vi "2.Rtde.vi"() -> ()   [LabVIEW 2023]
uses:
  UnderAutomation.UniversalRobots/UnderAutomation.UniversalRobots.lvlib
  C:/Users/fg/Documents/UniversalRobots.vi/LabVIEW_2024/UnderAutomation.UniversalRobots/lib/UnderAutomation.UniversalRobots.dll
  LabVIEW_2024/UnderAutomation.UniversalRobots/lib/UnderAutomation.UniversalRobots.dll
panel:
  out "Rtde":refnum<k24>
  out "UR Robot":refnum<k24>
  out "Connected":bool
  in  "Tab Control":enum32{"Connect to robot", "RTDE data"}(tab)
  in  "Disconnect":bool
  in  "Test":bool
  in  "Key":string
  in  "Licensee":string
  in  "Connect":bool
  in  "IP":string caption="Robot IP Address"
  out "License state":string
  out "Connect error":string
  in  "Speed":dbl(slide) scale=0.0..1.0 scale format="%#_2f"
  out "ActualTcpPose":T1
  out "TargetTcpSpeed":T1
  out "ScriptControlLine":u32
  out "OutputDoubleRegisters.X10":dbl
  out "OutputIntRegisters.X3":i32
  out "OutputIntRegisters.X2":i32
  out "OutputDoubleRegisters.X11":dbl
  out "OutputBitRegisters.X64":bool
  in  "InputIntRegisters.X11":i32
  in  "InputIntRegisters.X10":i32
  in  "Write":bool
  in  "stop":bool
  # "UnderAutomation"
  # "https://underautomation.com/universal-robots"
  # "+"
  # "LabVIEW demo app for remote control and monitoring of your Universal Robots cobot"
  # "Connect to robot"
  # "2. Ensure you have a trial or lifetime valid license"
  # "1. Set UR cobot address"
  # "This is a commercial library, you have a 30-day trial period. But you can use it forever if you buy a perpetual licence for your company (regardless of the number of robot, applications or developers)."
  # "If you have a license :"
  # "2. Connect to the robot"
  # "Output data received from robot"
  # "Output data received from robot"
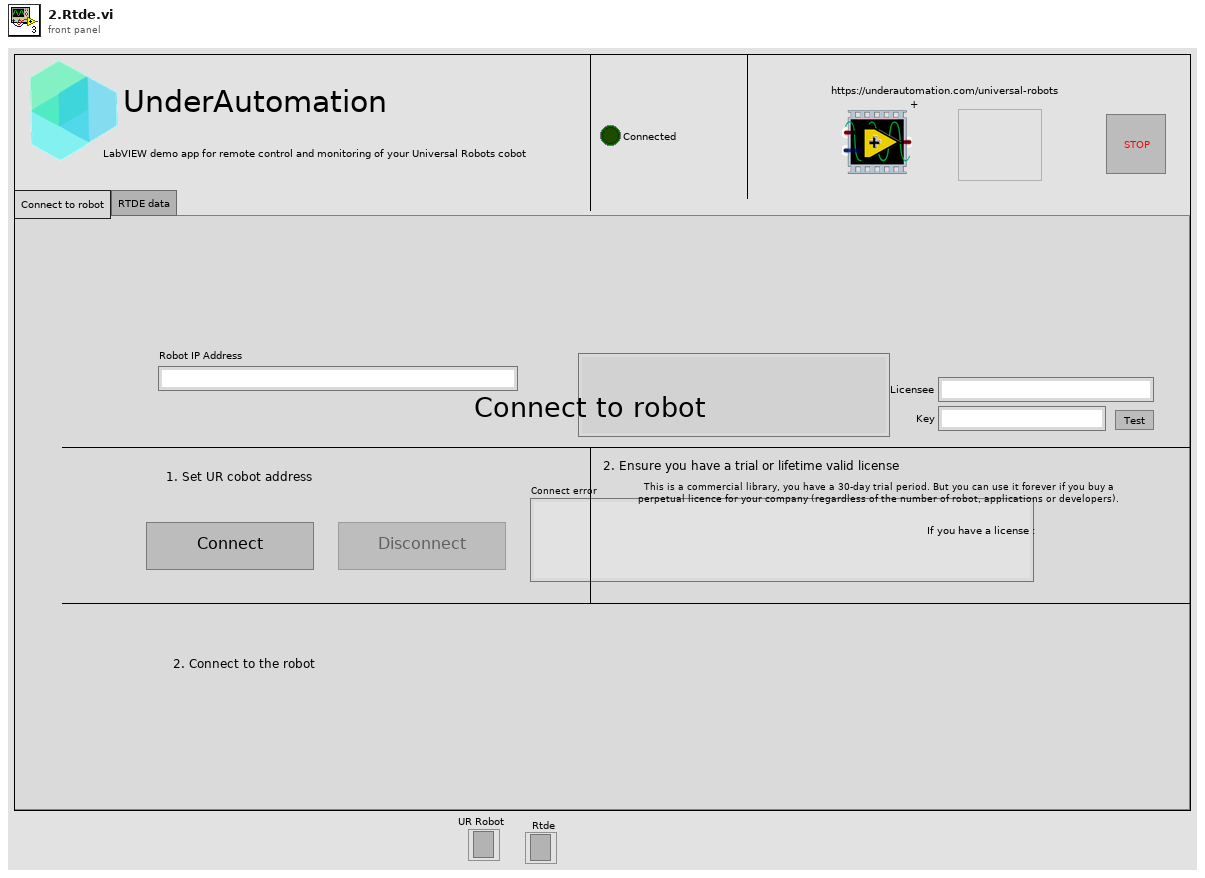
[diagram p1: front panel]
types:
  T1 = cluster{"X":dbl, "Y":dbl, "Z":dbl, "Rx":dbl, "Ry":dbl, "Rz":dbl}
  T2 = cluster{"ConfigurableDigitalOutput":u8, "ConfigurableDigitalOutputMask":u8, "ExternalForceTorque":cluster{"X":dbl, "Y":dbl, "Z":dbl, "Rx":dbl, "Ry":dbl, "Rz":dbl}, "InputBitRegisters":cluster{"X64":bool, "X65":bool, "X66":bool, "X67":bool, "X68":bool, "X69":bool, "X70":bool, "X71":bool, "X72":bool, "X73":bool, "X74":bool, "X75":bool, "X76":bool, "X77":bool, "X78":bool, "X79":bool, "X80":bool, "X81":bool, "X82":bool, "X83":bool, "X84":bool, "X85":bool, "X86":bool, "X87":bool, "X88":bool, "X89":bool, "X90":bool, "X91":bool, "X92":bool, "X93":bool, "X94":bool, "X95":bool, "X96":bool, "X97":bool, "X98":bool, "X99":bool, "X100":bool, "X101":bool, "X102":bool, "X103":bool, "X104":bool, "X105":bool, "X106":bool, "X107":bool, "X108":bool, "X109":bool, "X110":bool, "X111":bool, "X112":bool, "X113":bool, "X114":bool, "X115":bool, "X116":bool, "X117":bool, "X118":bool, "X119":bool, "X120":bool, "X121":bool, "X122":bool, "X123":bool, "X124":bool, "X125":bool, "X126":bool, "X127":bool}, "InputBtRegisters0To31":u32, "InputBtRegisters32To63":u32, "InputDoubleRegisters":cluster{"X0":dbl, "X1":dbl, "X2":dbl, "X3":dbl, "X4":dbl, "X5":dbl, "X6":dbl, "X7":dbl, "X8":dbl, "X9":dbl, "X10":dbl, "X11":dbl, "X12":dbl, "X13":dbl, "X14":dbl, "X15":dbl, "X16":dbl, "X17":dbl, "X18":dbl, "X19":dbl, "X20":dbl, "X21":dbl, "X22":dbl, "X23":dbl, "X24":dbl, "X25":dbl, "X26":dbl, "X27":dbl, "X28":dbl, "X29":dbl, "X30":dbl, "X31":dbl, "X32":dbl, "X33":dbl, "X34":dbl, "X35":dbl, "X36":dbl, "X37":dbl, "X38":dbl, "X39":dbl, "X40":dbl, "X41":dbl, "X42":dbl, "X43":dbl, "X44":dbl, "X45":dbl, "X46":dbl, "X47":dbl}, "InputIntRegisters":cluster{"X0":i32, "X1":i32, "X2":i32, "X3":i32, "X4":i32, "X5":i32, "X6":i32, "X7":i32, "X8":i32, "X9":i32, "X10":i32, "X11":i32, "X12":i32, "X13":i32, "X14":i32, "X15":i32, "X16":i32, "X17":i32, "X18":i32, "X19":i32, "X20":i32, "X21":i32, "X22":i32, "X23":i32, "X24":i32, "X25":i32, "X26":i32, "X27":i32, "X28":i32, "X29":i32, "X30":i32, "X31":i32, "X32":i32, "X33":i32, "X34":i32, "X35":i32, "X36":i32, "X37":i32, "X38":i32, "X39":i32, "X40":i32, "X41":i32, "X42":i32, "X43":i32, "X44":i32, "X45":i32, "X46":i32, "X47":i32}, "SpeedSliderFraction":dbl, "SpeedSliderMask":u32, "StandardAnalogOutput0":dbl, "StandardAnalogOutput1":dbl, "StandardAnalogOutputMask":u8, "StandardAnalogOutputType":u8, "StandardDigitalOutput":u8, "StandardDigitalOutputMask":u8}
  T3 = enum8{"Enabled", "Disabled", "Disabled and Grayed Out"}
  T4 = cluster{"ActualCurrent":cluster{"Base":dbl, "Elbow":dbl, "Shoulder":dbl, "Wrist1":dbl, "Wrist2":dbl, "Wrist3":dbl}, "ActualDigitalInputBits":u64, "ActualDigitalOutputBits":u64, "ActualExecutionTime":dbl, "ActualJointVoltage":cluster{"Base":dbl, "Elbow":dbl, "Shoulder":dbl, "Wrist1":dbl, "Wrist2":dbl, "Wrist3":dbl}, "ActualMainVoltage":dbl, "ActualMomentum":dbl, "ActualQ":cluster{"Base":dbl, "Elbow":dbl, "Shoulder":dbl, "Wrist1":dbl, "Wrist2":dbl, "Wrist3":dbl}, "ActualQd":cluster{"Base":dbl, "Elbow":dbl, "Shoulder":dbl, "Wrist1":dbl, "Wrist2":dbl, "Wrist3":dbl}, "ActualRobotCurrent":dbl, "ActualRobotVoltage":dbl, "ActualTcpForce":cluster{"X":dbl, "Y":dbl, "Z":dbl, "Rx":dbl, "Ry":dbl, "Rz":dbl}, "ActualTcpPose":cluster{"X":dbl, "Y":dbl, "Z":dbl, "Rx":dbl, "Ry":dbl, "Rz":dbl}, "ActualTcpSpeed":cluster{"X":dbl, "Y":dbl, "Z":dbl, "Rx":dbl, "Ry":dbl, "Rz":dbl}, "ActualToolAccelerometer":cluster{"X":dbl, "Y":dbl, "Z":dbl}, "AnalogIOTypes":u32, "ElbowPosition":cluster{"X":dbl, "Y":dbl, "Z":dbl}, "ElbowVelocity":cluster{"X":dbl, "Y":dbl, "Z":dbl}, "Euromap67_24VCurrent":dbl, "Euromap67_24VVoltage":dbl, "Euromap67InputBits":u32, "Euromap67OutputBits":u32, "FTRawWrench":cluster{"X":dbl, "Y":dbl, "Z":dbl, "Rx":dbl, "Ry":dbl, "Rz":dbl}, "InputBitRegisters":cluster{"X64":bool, "X65":bool, "X66":bool, "X67":bool, "X68":bool, "X69":bool, "X70":bool, "X71":bool, "X72":bool, "X73":bool, "X74":bool, "X75":bool, "X76":bool, "X77":bool, "X78":bool, "X79":bool, "X80":bool, "X81":bool, "X82":bool, "X83":bool, "X84":bool, "X85":bool, "X86":bool, "X87":bool, "X88":bool, "X89":bool, "X90":bool, "X91":bool, "X92":bool, "X93":bool, "X94":bool, "X95":bool, "X96":bool, "X97":bool, "X98":bool, "X99":bool, "X100":bool, "X101":bool, "X102":bool, "X103":bool, "X104":bool, "X105":bool, "X106":bool, "X107":bool, "X108":bool, "X109":bool, "X110":bool, "X111":bool, "X112":bool, "X113":bool, "X114":bool, "X115":bool, "X116":bool, "X117":bool, "X118":bool, "X119":bool, "X120":bool, "X121":bool, "X122":bool, "X123":bool, "X124":bool, "X125":bool, "X126":bool, "X127":bool}, "InputBitRegisters0To31":u32, "InputBitRegisters32To63":u32, "InputDoubleRegisters":cluster{"X0":dbl, "X1":dbl, "X2":dbl, "X3":dbl, "X4":dbl, "X5":dbl, "X6":dbl, "X7":dbl, "X8":dbl, "X9":dbl, "X10":dbl, "X11":dbl, "X12":dbl, "X13":dbl, "X14":dbl, "X15":dbl, "X16":dbl, "X17":dbl, "X18":dbl, "X19":dbl, "X20":dbl, "X21":dbl, "X22":dbl, "X23":dbl, "X24":dbl, "X25":dbl, "X26":dbl, "X27":dbl, "X28":dbl, "X29":dbl, "X30":dbl, "X31":dbl, "X32":dbl, "X33":dbl, "X34":dbl, "X35":dbl, "X36":dbl, "X37":dbl, "X38":dbl, "X39":dbl, "X40":dbl, "X41":dbl, "X42":dbl, "X43":dbl, "X44":dbl, "X45":dbl, "X46":dbl, "X47":dbl}, "InputIntRegisters":cluster{"X0":i32, "X1":i32, "X2":i32, "X3":i32, "X4":i32, "X5":i32, "X6":i32, "X7":i32, "X8":i32, "X9":i32, "X10":i32, "X11":i32, "X12":i32, "X13":i32, "X14":i32, "X15":i32, "X16":i32, "X17":i32, "X18":i32, "X19":i32, "X20":i32, "X21":i32, "X22":i32, "X23":i32, "X24":i32, "X25":i32, "X26":i32, "X27":i32, "X28":i32, "X29":i32, "X30":i32, "X31":i32, "X32":i32, "X33":i32, "X34":i32, "X35":i32, "X36":i32, "X37":i32, "X38":i32, "X39":i32, "X40":i32, "X41":i32, "X42":i32, "X43":i32, "X44":i32, "X45":i32, "X46":i32, "X47":i32}, "IOCurrent":dbl, "JointControlOutput":cluster{"Base":dbl, "Elbow":dbl, "Shoulder":dbl, "Wrist1":dbl, "Wrist2":dbl, "Wrist3":dbl}, "JointMode":cluster{"Base":i32, "Elbow":i32, "Shoulder":i32, "Wrist1":i32, "Wrist2":i32, "Wrist3":i32}, "JointTemperatures":cluster{"Base":dbl, "Elbow":dbl, "Shoulder":dbl, "Wrist1":dbl, "Wrist2":dbl, "Wrist3":dbl}, "OutputBitRegisters":cluster{"X64":bool, "X65":bool, "X66":bool, "X67":bool, "X68":bool, "X69":bool, "X70":bool, "X71":bool, "X72":bool, "X73":bool, "X74":bool, "X75":bool, "X76":bool, "X77":bool, "X78":bool, "X79":bool, "X80":bool, "X81":bool, "X82":bool, "X83":bool, "X84":bool, "X85":bool, "X86":bool, "X87":bool, "X88":bool, "X89":bool, "X90":bool, "X91":bool, "X92":bool, "X93":bool, "X94":bool, "X95":bool, "X96":bool, "X97":bool, "X98":bool, "X99":bool, "X100":bool, "X101":bool, "X102":bool, "X103":bool, "X104":bool, "X105":bool, "X106":bool, "X107":bool, "X108":bool, "X109":bool, "X110":bool, "X111":bool, "X112":bool, "X113":bool, "X114":bool, "X115":bool, "X116":bool, "X117":bool, "X118":bool, "X119":bool, "X120":bool, "X121":bool, "X122":bool, "X123":bool, "X124":bool, "X125":bool, "X126":bool, "X127":bool}, "OutputBitRegisters0To31":u32, "OutputBitRegisters32To63":u32, "OutputDoubleRegisters":cluster{"X0":dbl, "X1":dbl, "X2":dbl, "X3":dbl, "X4":dbl, "X5":dbl, "X6":dbl, "X7":dbl, "X8":dbl, "X9":dbl, "X10":dbl, "X11":dbl, "X12":dbl, "X13":dbl, "X14":dbl, "X15":dbl, "X16":dbl, "X17":dbl, "X18":dbl, "X19":dbl, "X20":dbl, "X21":dbl, "X22":dbl, "X23":dbl, "X24":dbl, "X25":dbl, "X26":dbl, "X27":dbl, "X28":dbl, "X29":dbl, "X30":dbl, "X31":dbl, "X32":dbl, "X33":dbl, "X34":dbl, "X35":dbl, "X36":dbl, "X37":dbl, "X38":dbl, "X39":dbl, "X40":dbl, "X41":dbl, "X42":dbl, "X43":dbl, "X44":dbl, "X45":dbl, "X46":dbl, "X47":dbl}, "OutputIntRegisters":cluster{"X0":i32, "X1":i32, "X2":i32, "X3":i32, "X4":i32, "X5":i32, "X6":i32, "X7":i32, "X8":i32, "X9":i32, "X10":i32, "X11":i32, "X12":i32, "X13":i32, "X14":i32, "X15":i32, "X16":i32, "X17":i32, "X18":i32, "X19":i32, "X20":i32, "X21":i32, "X22":i32, "X23":i32, "X24":i32, "X25":i32, "X26":i32, "X27":i32, "X28":i32, "X29":i32, "X30":i32, "X31":i32, "X32":i32, "X33":i32, "X34":i32, "X35":i32, "X36":i32, "X37":i32, "X38":i32, "X39":i32, "X40":i32, "X41":i32, "X42":i32, "X43":i32, "X44":i32, "X45":i32, "X46":i32, "X47":i32}, "Payload":dbl, "PayloadCOG":cluster{"X":dbl, "Y":dbl, "Z":dbl}, "PayloadInertia":cluster{"X":dbl, "Y":dbl, "Z":dbl, "Rx":dbl, "Ry":dbl, "Rz":dbl}, "RobotMode":i32, "RobotStatusBits":u32, "RuntimeState":u32, "SafetyMode":i32, "SafetyStatus":i32, "SafetyStatusBits":u32, "ScriptControlLine":u32, "SpeedScaling":dbl, "StandardAnalogInput0":dbl, "StandardAnalogInput1":dbl, "StandardAnalogOutput0":dbl, "StandardAnalogOutput1":dbl, "TargetCurrent":cluster{"Base":dbl, "Elbow":dbl, "Shoulder":dbl, "Wrist1":dbl, "Wrist2":dbl, "Wrist3":dbl}, "TargetMoment":cluster{"Base":dbl, "Elbow":dbl, "Shoulder":dbl, "Wrist1":dbl, "Wrist2":dbl, "Wrist3":dbl}, "TargetQ":cluster{"Base":dbl, "Elbow":dbl, "Shoulder":dbl, "Wrist1":dbl, "Wrist2":dbl, "Wrist3":dbl}, "TargetQd":cluster{"Base":dbl, "Elbow":dbl, "Shoulder":dbl, "Wrist1":dbl, "Wrist2":dbl, "Wrist3":dbl}, "TargetQdd":cluster{"Base":dbl, "Elbow":dbl, "Shoulder":dbl, "Wrist1":dbl, "Wrist2":dbl, "Wrist3":dbl}, "TargetSpeedFraction":dbl, "TargetTcpPose":cluster{"X":dbl, "Y":dbl, "Z":dbl, "Rx":dbl, "Ry":dbl, "Rz":dbl}, "TargetTcpSpeed":cluster{"X":dbl, "Y":dbl, "Z":dbl, "Rx":dbl, "Ry":dbl, "Rz":dbl}, "TcpForceScalar":dbl, "Timestamp":dbl, "ToolAnalogInput0":dbl, "ToolAnalogInput1":dbl, "ToolAnalogInputTypes":u32, "ToolDigitalOutput0mode":u8, "ToolDigitalOutput1Mode":u8, "ToolMode":u32, "ToolOutputCurrent":dbl, "ToolOutputMode":u8, "ToolOutputVoltage":i32, "ToolTemperature":dbl}
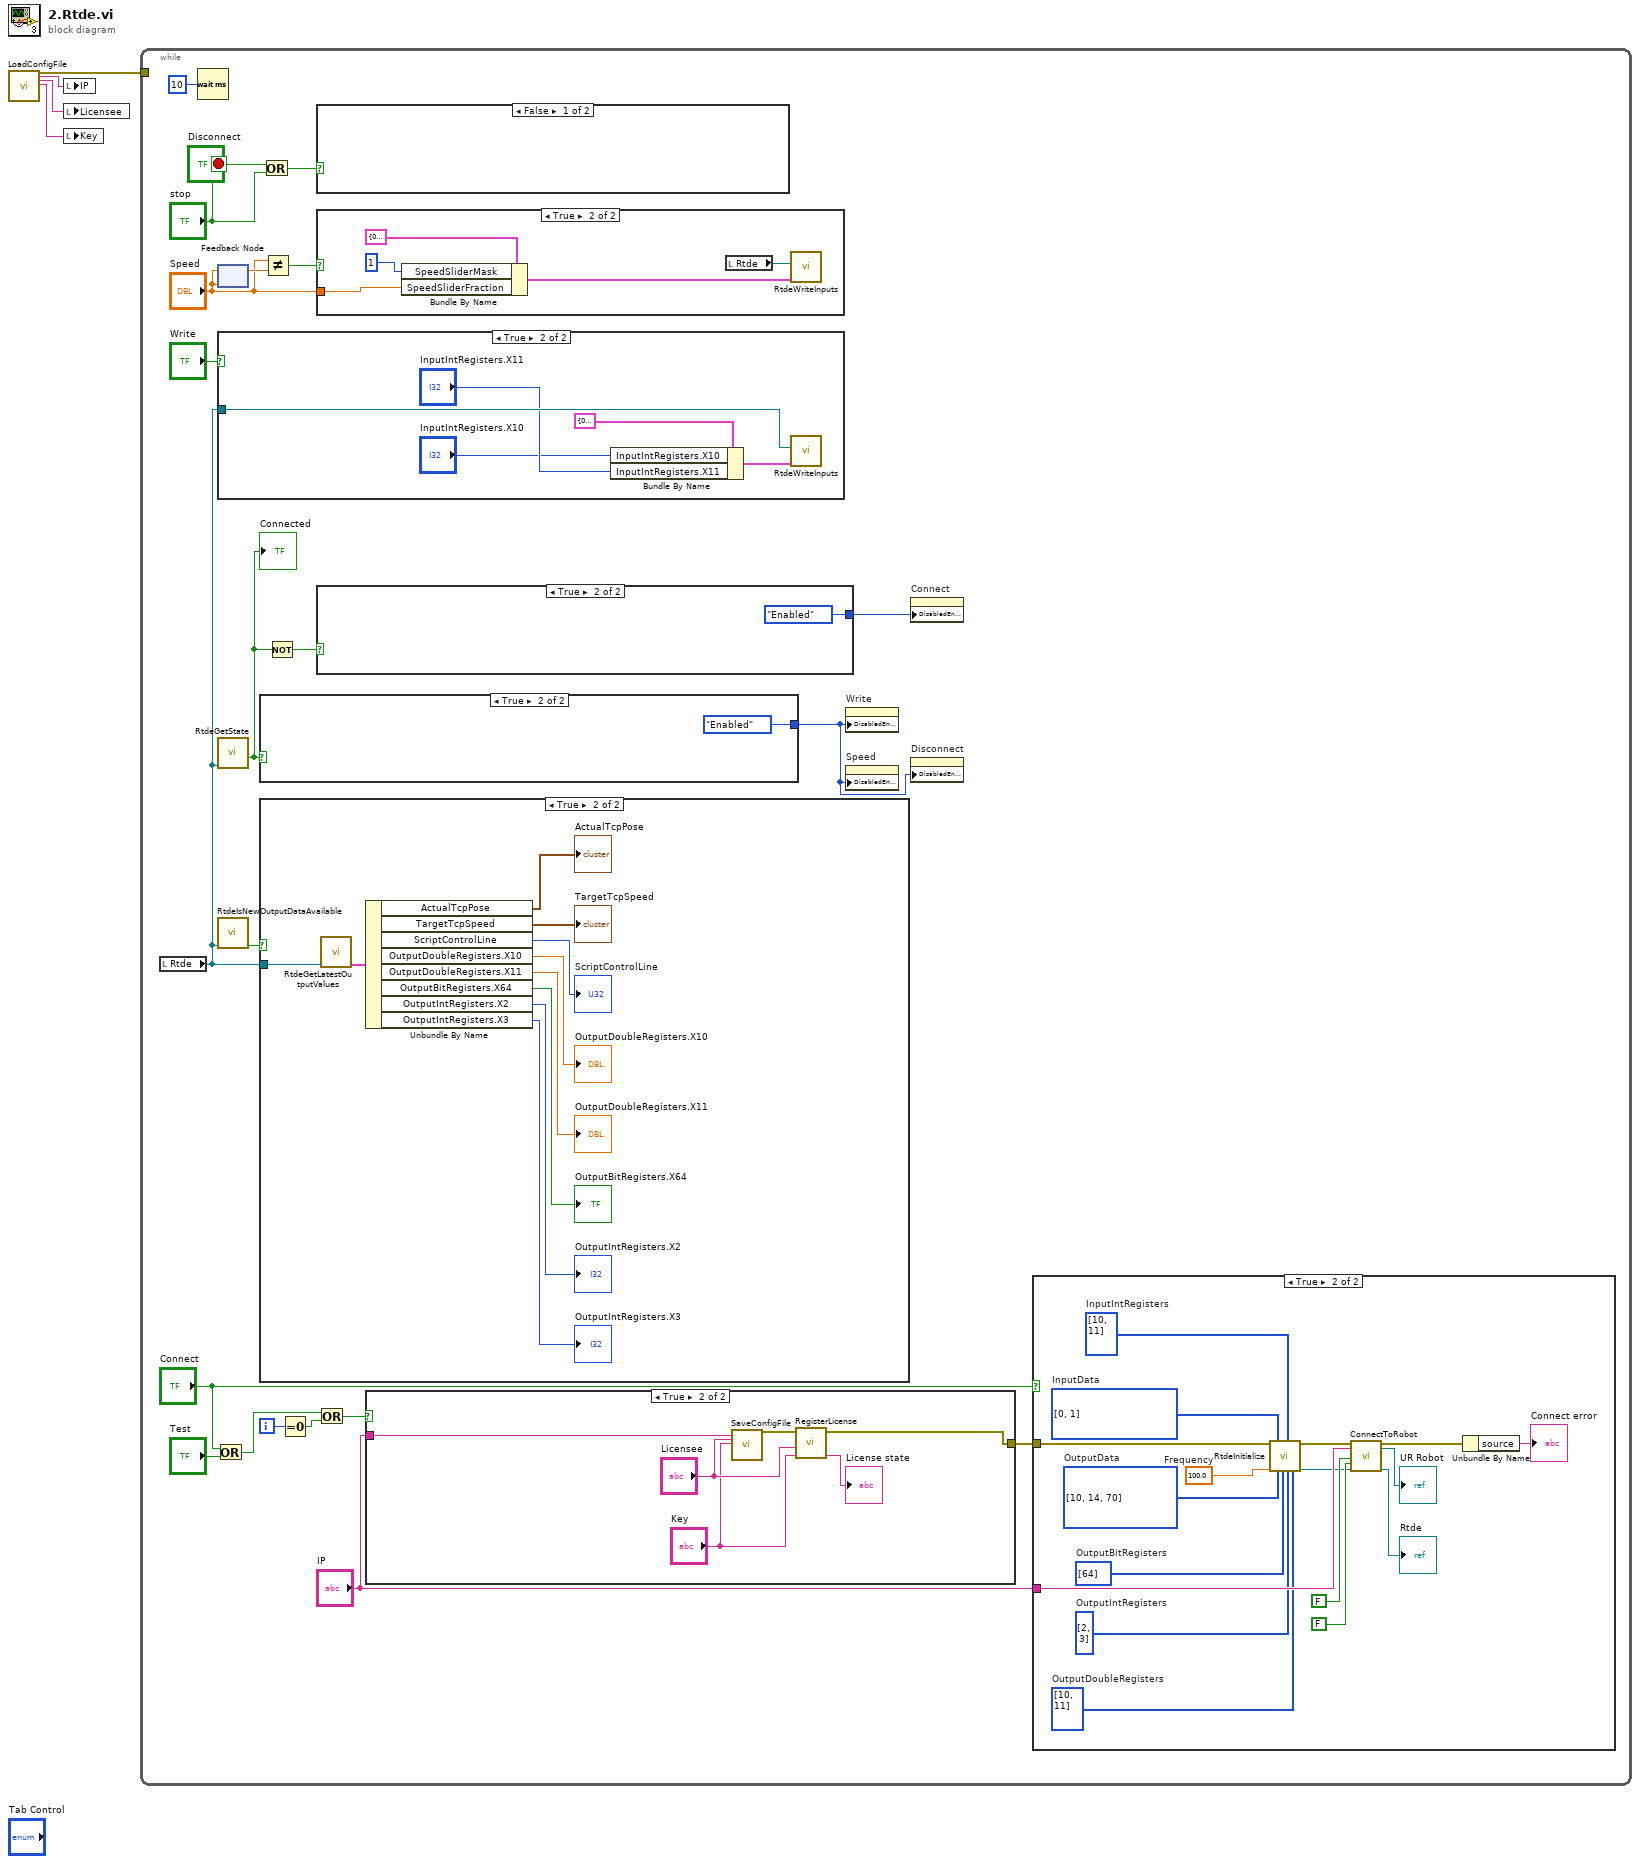
[diagram p0: block diagram]
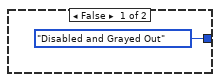
[diagram p5: hidden frame]
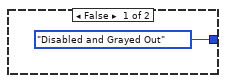
[diagram p6: hidden frame]
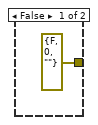
[diagram p7: hidden frame]
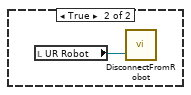
[diagram p9: hidden frame]
diagram:
  n1 = call "LoadConfigFile.vi"() -> ("error out"=w1:errorcluster, "IP"=w2:string, "Licensee"=w4:string, "Key"=w3:string)  [unwired: 22 in, 2 out]
  n2 = local write "IP"(w2) -> ()
  n3 = local write "Licensee"(w4) -> ()
  n4 = local write "Key"(w3) -> ()
  n5 = while {
    tunnel: w1 -> [_]
    i -> [w21]
    stop <- "stop" stop-if-true
    n6 = local read "Rtde"() -> (w10:refnum<k24>)
    n7 = Wait (ms)(milliseconds to wait=u32 10) -> ()  [unwired: 1 out]
    n8 = Or(x="Connect", y="Test") -> (x .or. y?=w19:bool)
    n9 = feedback #1("Speed") -> (w8:dbl)
    n10 = feedback-in #1("Speed") -> ()
    n11 = case shown="True" "Write" {
      tunnel: w10 -> [_ w36]
      frame False {
      }
      frame True {
        n12 = Bundle By Name(cluster=T2 {"ConfigurableDigitalOutput"=0, "ConfigurableDigitalOutputMask"=0, "ExternalForceTorque"={"X"=0.0, "Y"=0.0, "Z"=0.0, "Rx"=0.0, "Ry"=0.0, "Rz"=0.0}, "InputBitRegisters"={"X64"=FALSE, "X65"=FALSE, "X66"=FALSE, "X67"=FALSE, "X68"=FALSE, "X69"=FALSE, "X70"=FALSE, "X71"=FALSE, "X72"=FALSE, "X73"=FALSE, "X74"=FALSE, "X75"=FALSE, "X76"=FALSE, "X77"=FALSE, "X78"=FALSE, "X79"=FALSE, "X80"=FALSE, "X81"=FALSE, "X82"=FALSE, "X83"=FALSE, "X84"=FALSE, "X85"=FALSE, "X86"=FALSE, "X87"=FALSE, "X88"=FALSE, "X89"=FALSE, "X90"=FALSE, "X91"=FALSE, "X92"=FALSE, "X93"=FALSE, "X94"=FALSE, "X95"=FALSE, "X96"=FALSE, "X97"=FALSE, "X98"=FALSE, "X99"=FALSE, "X100"=FALSE, "X101"=FALSE, "X102"=FALSE, "X103"=FALSE, "X104"=FALSE, "X105"=FALSE, "X106"=FALSE, "X107"=FALSE, "X108"=FALSE, "X109"=FALSE, "X110"=FALSE, "X111"=FALSE, "X112"=FALSE, "X113"=FALSE, "X114"=FALSE, "X115"=FALSE, "X116"=FALSE, "X117"=FALSE, "X118"=FALSE, "X119"=FALSE, "X120"=FALSE, "X121"=FALSE, "X122"=FALSE, "X123"=FALSE, "X124"=FALSE, "X125"=FALSE, "X126"=FALSE, "X127"=FALSE}, "InputBtRegisters0To31"=0, "InputBtRegisters32To63"=0, "InputDoubleRegisters"={"X0"=0.0, "X1"=0.0, "X2"=0.0, "X3"=0.0, "X4"=0.0, "X5"=0.0, "X6"=0.0, "X7"=0.0, "X8"=0.0, "X9"=0.0, "X10"=0.0, "X11"=0.0, "X12"=0.0, "X13"=0.0, "X14"=0.0, "X15"=0.0, "X16"=0.0, "X17"=0.0, "X18"=0.0, "X19"=0.0, "X20"=0.0, "X21"=0.0, "X22"=0.0, "X23"=0.0, "X24"=0.0, "X25"=0.0, "X26"=0.0, "X27"=0.0, "X28"=0.0, "X29"=0.0, "X30"=0.0, "X31"=0.0, "X32"=0.0, "X33"=0.0, "X34"=0.0, "X35"=0.0, "X36"=0.0, "X37"=0.0, "X38"=0.0, "X39"=0.0, "X40"=0.0, "X41"=0.0, "X42"=0.0, "X43"=0.0, "X44"=0.0, "X45"=0.0, "X46"=0.0, "X47"=0.0}, "InputIntRegisters"={"X0"=0, "X1"=0, "X2"=0, "X3"=0, "X4"=0, "X5"=0, "X6"=0, "X7"=0, "X8"=0, "X9"=0, "X10"=0, "X11"=0, "X12"=0, "X13"=0, "X14"=0, "X15"=0, "X16"=0, "X17"=0, "X18"=0, "X19"=0, "X20"=0, "X21"=0, "X22"=0, "X23"=0, "X24"=0, "X25"=0, "X26"=0, "X27"=0, "X28"=0, "X29"=0, "X30"=0, "X31"=0, "X32"=0, "X33"=0, "X34"=0, "X35"=0, "X36"=0, "X37"=0, "X38"=0, "X39"=0, "X40"=0, "X41"=0, "X42"=0, "X43"=0, "X44"=0, "X45"=0, "X46"=0, "X47"=0}, "SpeedSliderFraction"=0.0, "SpeedSliderMask"=0, "StandardAnalogOutput0"=0.0, "StandardAnalogOutput1"=0.0, "StandardAnalogOutputMask"=0, "StandardAnalogOutputType"=0, "StandardDigitalOutput"=0, "StandardDigitalOutputMask"=0} ("Data"), "InputIntRegisters.X10"="InputIntRegisters.X10", "InputIntRegisters.X11"="InputIntRegisters.X11") -> (w35:T2)
        n13 = call "RtdeWriteInputs.vi"("Data"=w35, "Rtde"=w36) -> ()  [unwired: 9 in, 1 out]
      }
    }
    n14 = call "RtdeGetState.vi"("Rtde"=w10) -> ("Connected"=w13:bool)  [unwired: 8 in, 2 out]
    "Connected" <- w13
    n15 = call "RtdeIsNewOutputDataAvailable.vi"("Rtde"=w10) -> ("Data available"=w12:bool)  [unwired: 9 in, 1 out]
    n16 = case shown="True" w13 {
      tunnel: [T3."Disabled and Grayed Out" ("Disabled") T3."Enabled" ("Disabled")] -> w5
      frame False {
      }
      frame True {
      }
    }
    n17 = case shown="True" w12 {
      tunnel: w10 -> [_ w46]
      frame False {
      }
      frame True {
        n18 = call "RtdeGetLatestOutputValues.vi"("Rtde"=w46) -> ("Data"=w45:T4)  [unwired: 9 in, 1 out]
        n19 = Unbundle By Name(w45) -> ("ActualTcpPose"=→"ActualTcpPose":T1, "TargetTcpSpeed"=→"TargetTcpSpeed":T1, "ScriptControlLine"=→"ScriptControlLine":u32, "OutputDoubleRegisters.X10"=→"OutputDoubleRegisters.X10":dbl, "OutputDoubleRegisters.X11"=→"OutputDoubleRegisters.X11":dbl, "OutputBitRegisters.X64"=→"OutputBitRegisters.X64":bool, "OutputIntRegisters.X2"=→"OutputIntRegisters.X2":i32, "OutputIntRegisters.X3"=→"OutputIntRegisters.X3":i32)
      }
    }
    n20 = Or(x="Disconnect", y="stop") -> (x .or. y?=w24:bool)
    n21 = Not Equal?(x="Speed", y=w8) -> (x != y?=w7:bool)
    n22 = Not(x=w13) -> (.not. x?=w15:bool)
    n23 = Equal To 0?(x=w21) -> (x = 0?=w20:bool)
    n24 = case shown="False" w24 {
      frame False {
      }
      frame True {
        n25 = local read "UR Robot"() -> (w75:refnum<k24>)
        n26 = call "DisconnectFromRobot.vi"("UR Robot"=w75) -> ()  [unwired: 2 in, 1 out]
      }
    }
    n27 = case shown="True" w7 {
      tunnel: "Speed" -> [_ w27]
      frame False {
      }
      frame True {
        n28 = Bundle By Name(cluster=T2 {"ConfigurableDigitalOutput"=0, "ConfigurableDigitalOutputMask"=0, "ExternalForceTorque"={"X"=0.0, "Y"=0.0, "Z"=0.0, "Rx"=0.0, "Ry"=0.0, "Rz"=0.0}, "InputBitRegisters"={"X64"=FALSE, "X65"=FALSE, "X66"=FALSE, "X67"=FALSE, "X68"=FALSE, "X69"=FALSE, "X70"=FALSE, "X71"=FALSE, "X72"=FALSE, "X73"=FALSE, "X74"=FALSE, "X75"=FALSE, "X76"=FALSE, "X77"=FALSE, "X78"=FALSE, "X79"=FALSE, "X80"=FALSE, "X81"=FALSE, "X82"=FALSE, "X83"=FALSE, "X84"=FALSE, "X85"=FALSE, "X86"=FALSE, "X87"=FALSE, "X88"=FALSE, "X89"=FALSE, "X90"=FALSE, "X91"=FALSE, "X92"=FALSE, "X93"=FALSE, "X94"=FALSE, "X95"=FALSE, "X96"=FALSE, "X97"=FALSE, "X98"=FALSE, "X99"=FALSE, "X100"=FALSE, "X101"=FALSE, "X102"=FALSE, "X103"=FALSE, "X104"=FALSE, "X105"=FALSE, "X106"=FALSE, "X107"=FALSE, "X108"=FALSE, "X109"=FALSE, "X110"=FALSE, "X111"=FALSE, "X112"=FALSE, "X113"=FALSE, "X114"=FALSE, "X115"=FALSE, "X116"=FALSE, "X117"=FALSE, "X118"=FALSE, "X119"=FALSE, "X120"=FALSE, "X121"=FALSE, "X122"=FALSE, "X123"=FALSE, "X124"=FALSE, "X125"=FALSE, "X126"=FALSE, "X127"=FALSE}, "InputBtRegisters0To31"=0, "InputBtRegisters32To63"=0, "InputDoubleRegisters"={"X0"=0.0, "X1"=0.0, "X2"=0.0, "X3"=0.0, "X4"=0.0, "X5"=0.0, "X6"=0.0, "X7"=0.0, "X8"=0.0, "X9"=0.0, "X10"=0.0, "X11"=0.0, "X12"=0.0, "X13"=0.0, "X14"=0.0, "X15"=0.0, "X16"=0.0, "X17"=0.0, "X18"=0.0, "X19"=0.0, "X20"=0.0, "X21"=0.0, "X22"=0.0, "X23"=0.0, "X24"=0.0, "X25"=0.0, "X26"=0.0, "X27"=0.0, "X28"=0.0, "X29"=0.0, "X30"=0.0, "X31"=0.0, "X32"=0.0, "X33"=0.0, "X34"=0.0, "X35"=0.0, "X36"=0.0, "X37"=0.0, "X38"=0.0, "X39"=0.0, "X40"=0.0, "X41"=0.0, "X42"=0.0, "X43"=0.0, "X44"=0.0, "X45"=0.0, "X46"=0.0, "X47"=0.0}, "InputIntRegisters"={"X0"=0, "X1"=0, "X2"=0, "X3"=0, "X4"=0, "X5"=0, "X6"=0, "X7"=0, "X8"=0, "X9"=0, "X10"=0, "X11"=0, "X12"=0, "X13"=0, "X14"=0, "X15"=0, "X16"=0, "X17"=0, "X18"=0, "X19"=0, "X20"=0, "X21"=0, "X22"=0, "X23"=0, "X24"=0, "X25"=0, "X26"=0, "X27"=0, "X28"=0, "X29"=0, "X30"=0, "X31"=0, "X32"=0, "X33"=0, "X34"=0, "X35"=0, "X36"=0, "X37"=0, "X38"=0, "X39"=0, "X40"=0, "X41"=0, "X42"=0, "X43"=0, "X44"=0, "X45"=0, "X46"=0, "X47"=0}, "SpeedSliderFraction"=0.0, "SpeedSliderMask"=0, "StandardAnalogOutput0"=0.0, "StandardAnalogOutput1"=0.0, "StandardAnalogOutputMask"=0, "StandardAnalogOutputType"=0, "StandardDigitalOutput"=0, "StandardDigitalOutputMask"=0} ("Data"), "SpeedSliderMask"=u32 1, "SpeedSliderFraction"=w27) -> (w30:T2)
        n29 = local read "Rtde"() -> (w31:refnum<k24>)
        n30 = call "RtdeWriteInputs.vi"("Data"=w30, "Rtde"=w31) -> ()  [unwired: 9 in, 1 out]
      }
    }
    n31 = case shown="True" w15 {
      tunnel: [T3."Disabled and Grayed Out" ("Disabled") T3."Enabled" ("Disabled")] -> w14
      frame False {
      }
      frame True {
      }
    }
    n32 = Or(x=w19, y=w20) -> (x .or. y?=w18:bool)
    n33 = case shown="True" w18 {
      tunnel: [errorcluster {"status"=FALSE, "code"=0, "source"=""} ("error out") w56] -> w17
      tunnel: "IP" -> [_ w53]
      frame False {
      }
      frame True {
        n34 = call "SaveConfigFile.vi"("IP"=w53, "Licensee"="Licensee", "Key"="Key") -> ("error out"=w52:errorcluster)  [unwired: 24 in]
        n35 = call "RegisterLicense.vi"("key"="Key", "licensee"="Licensee", "error in"=w52) -> ("State message"=→"License state":string, "error out"=w56:errorcluster)  [unwired: 5 in, 1 out]
      }
    }
    n36 = property on="Write" class="Bool"("DisabledEnum"=w5) -> ()  [unwired: 2 in, 2 out]
    n37 = property on="Speed" class="Slide (strict)"("DisabledEnum"=w5) -> ()  [unwired: 2 in, 2 out]
    n38 = property on="Connect" class="Bool"("DisabledEnum"=w14) -> ()  [unwired: 2 in, 2 out]
    n39 = property on="Disconnect" class="Bool"("DisabledEnum"=w5) -> ()  [unwired: 2 in, 2 out]
    n40 = case shown="True" "Connect" {
      tunnel: w17 -> [_ w62]
      tunnel: "IP" -> [_ w69]
      frame False {
      }
      frame True {
        w58 = i32[] [2, 3]  # OutputIntRegisters
        w59 = i32[] [64]  # OutputBitRegisters
        w60 = i32[] [10, 11]  # OutputDoubleRegisters
        w64 = i32[] [10, 11]  # InputIntRegisters
        w65 = i32[] [0, 1] items=["SpeedSliderMask", "SpeedSliderFraction", "StandardDigitalOutputMask", "ConfigurableDigitalOutputMask", "StandardDigitalOutput", "ConfigurableDigitalOutput", "StandardAnalogOutputMask", "StandardAnalogOutputType", "StandardAnalogOutput0", "StandardAnalogOutput1", "InputBtRegisters0To31", "InputBtRegisters32To63", "InputBitRegisters", "InputIntRegisters", "InputDoubleRegisters", "ExternalForceTorque"]  # InputData
        w66 = 100.0  # Frequency
        w67 = i32[] [10, 14, 70] items=["Timestamp", "TargetQ", "TargetQd", "TargetQdd", "TargetCurrent", "TargetMoment", "ActualQ", "ActualQd", "ActualCurrent", "JointControlOutput", "ActualTcpPose", "ActualTcpSpeed", "ActualTcpForce", "TargetTcpPose", "TargetTcpSpeed", "ActualDigitalInputBits", "JointTemperatures", "ActualExecutionTime", "RobotMode", "JointMode", "SafetyMode", "SafetyStatus", "ActualToolAccelerometer", "SpeedScaling", "TargetSpeedFraction", "ActualMomentum", "ActualMainVoltage", "ActualRobotVoltage", "ActualRobotCurrent", "ActualJointVoltage", "ActualDigitalOutputBits", "RuntimeState", "ElbowPosition", "ElbowVelocity", "RobotStatusBits", "SafetyStatusBits", "AnalogIOTypes", "StandardAnalogInput0", "StandardAnalogInput1", "StandardAnalogOutput0", "StandardAnalogOutput1", "IOCurrent", "Euromap67InputBits", "Euromap67OutputBits", "Euromap67_24VVoltage", "Euromap67_24VCurrent", "ToolMode", "ToolAnalogInputTypes", "ToolAnalogInput0", "ToolAnalogInput1", "ToolOutputVoltage", "ToolOutputCurrent", "ToolTemperature", "TcpForceScalar", "OutputBitRegisters0To31", "OutputBitRegisters32To63", "OutputBitRegisters", "OutputIntRegisters", "OutputDoubleRegisters", "InputBitRegisters0To31", "InputBitRegisters32To63", "InputBitRegisters", "InputIntRegisters", "InputDoubleRegisters", "ToolOutputMode", "ToolDigitalOutput0mode", "ToolDigitalOutput1Mode", "Payload", "PayloadCOG", "PayloadInertia", "ScriptControlLine", "FTRawWrench"]  # OutputData
        n41 = call "RtdeInitialize.vi"("error in"=w62, "Frequency"=w66, "InputData"=w65, "OutputData"=w67, "OutputBitRegisters"=w59, "InputIntRegisters"=w64, "OutputIntRegisters"=w58, "OutputDoubleRegisters"=w60) -> ("error out"=w61:errorcluster, "RTDE Connect Parameters"=w63:refnum<k24>)  [unwired: 10 in]
        n42 = call "ConnectToRobot.vi"("error in"=w61, "ip"=w69, "Enable Dashboard"=FALSE ("Enable Primary Interface"), "Enable Primary Interface"=FALSE, "RTDE Connect Parameters"=w63) -> ("error out"=w72:errorcluster, "UR Robot"=→"UR Robot":refnum<k24>, "Rtde"=→"Rtde":refnum<k24>)  [unwired: 9 in, 3 out]
        n43 = Unbundle By Name(w72) -> ("source"=→"Connect error":string)
      }
    }
  }
